vi "Write Sub Panel.vi"(8 "error in (no error)":errorcluster, 10 "Sub Panel":refnum<vi>, 11 "Items in":refnum<class "Items.lvclass">) -> (0 "error out":errorcluster, 3 "Items out":refnum<class "Items.lvclass">)   [LabVIEW 2020, in "Items.lvlib" / "Items.lvclass"]
uses:
  Items.lvclass
  Items.lvclass/Items.ctl
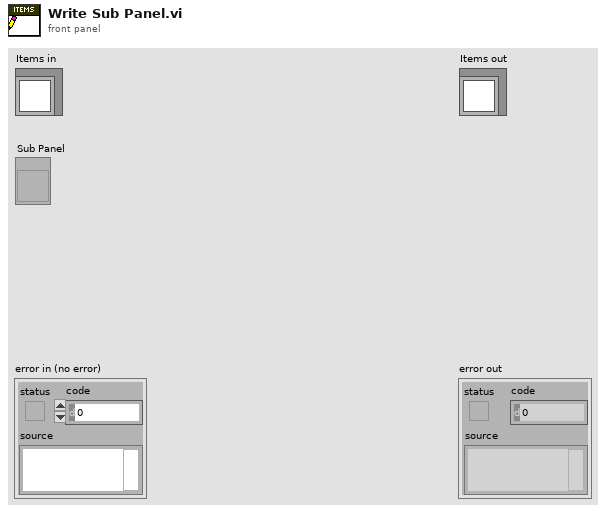
[diagram p1: front panel]
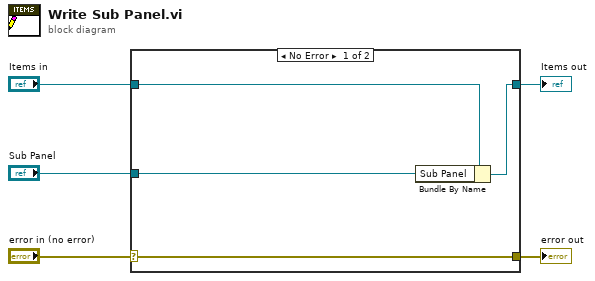
[diagram p0: block diagram]
diagram:
  n1 = case shown="No Error" "error in (no error)" {
    selector: "error in (no error)" -> [w9 w10]
    tunnel: [w9 w10] -> w4
    tunnel: [w7 w11] -> w2
    tunnel: "Items in" -> [w8 w11]
    tunnel: "Sub Panel" -> [w6 _]
    frame No Error {
      n2 = Bundle By Name(cluster=w8, "Sub Panel"=w6) -> (w7:refnum<class "Items.lvclass">)
    }
    frame Error {
    }
  }
  "error out" <- w4
  "Items out" <- w2
